vi "Read.vi"(0 "channel":T1, 1 "timeout in ms (0)":i32) -> (2 "missed":i32, 3 "element":T2)   [LabVIEW 2020]
doc: "Reads a value from a Tag channel."
uses:
  Element.ctl
  Flex.lvlib
  ))Channel.ctl
panel:
  # "number of values missed\n(-1 means element is stale)"
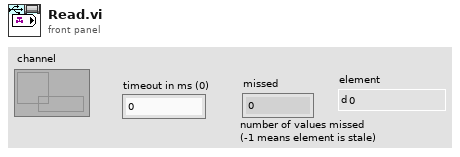
[diagram p1: front panel]
types:
  T1 = typedef "Flex.lvlib/))Channel.ctl" = refnum<queue>
  T2 = typedef "Flex.lvlib/Element.ctl" = dbl
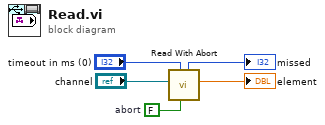
[diagram p0: block diagram]
diagram:
  w1 = FALSE  # abort
  n1 = call "Read With Abort.vi"("abort"=w1, "timeout in ms (0)"="timeout in ms (0)", "channel"="channel") -> ("element"=→"element":T2, "missed"=→"missed":i32)  [unwired: 6 in, 1 out]
